vi "Follower.vi"   [LabVIEW 2016]
uses:
  <vilib>/NXT/Block Support/NXT_InputPort.ctl
  <vilib>/NXT/Block Support/NXT_TimerIndex.ctl
  <vilib>/NXT/Block Support/NXT_OutputPort.ctl
  <vilib>/NXT/Dual Mode Library/Sensors/EV3_Color_Reflect.vi
  <vilib>/NXT/NXTIO Xnodes/NXTIONodeSubVIs/NXTStopMotors.vi
  <vilib>/NXT/Dual Mode Library/Sensors/EV3_Ultrasonic_CM.vi
  <vilib>/NXT/NXTIO Xnodes/NXTIONodeSubVIs/NXTMoveMotors.vi
  <vilib>/NXT/Dual Mode Library/Display/drawText_Right.vi
  <vilib>/NXT/Dual Mode Library/Display/drawNumber.vi
  <vilib>/NXT/Dual Mode Library/Display/drawNumber_float.vi
  <vilib>/NXT/Dual Mode Library/Sensors/Touch_Pressed.vi
  <vilib>/NXT/Dual Mode Library/Display/drawText.vi
  <vilib>/NXT/Subs/LVHSConnector.ctl
  <vilib>/NXT/NXTIO Xnodes/AddressXNode/NXTIOAddress.xnode
  <vilib>/NXT/NXTIO Xnodes/NXTIOXNode/NXTIO.xnode
  <vilib>/NXT/LegoClasses/BrickReference/BrickReference.lvclass
types:
  T1 = typedef "NXT_TimerIndex.ctl" = u8
  T2 = typedef "LVHSConnector.ctl" = refnum<class "BrickReference.lvclass">
  T3 = typedef "NXT_InputPort.ctl" = u32
  T4 = typedef "NXT_OutputPort.ctl" = u8
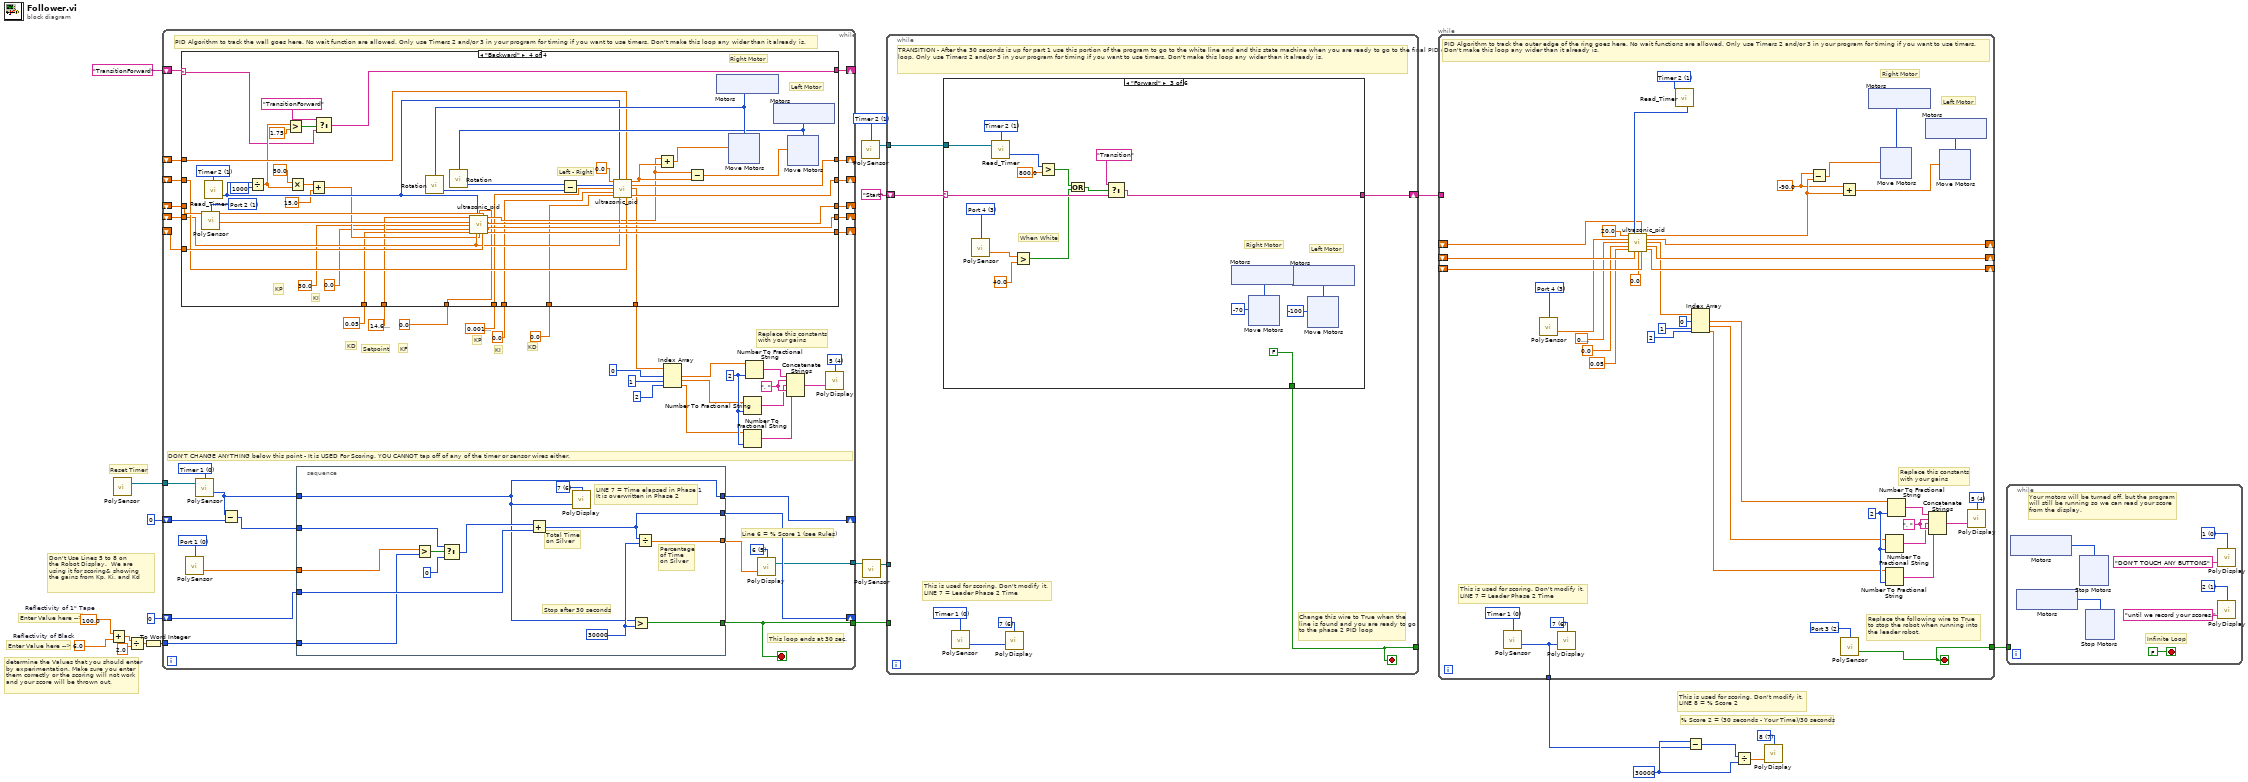
[diagram p0: block diagram]
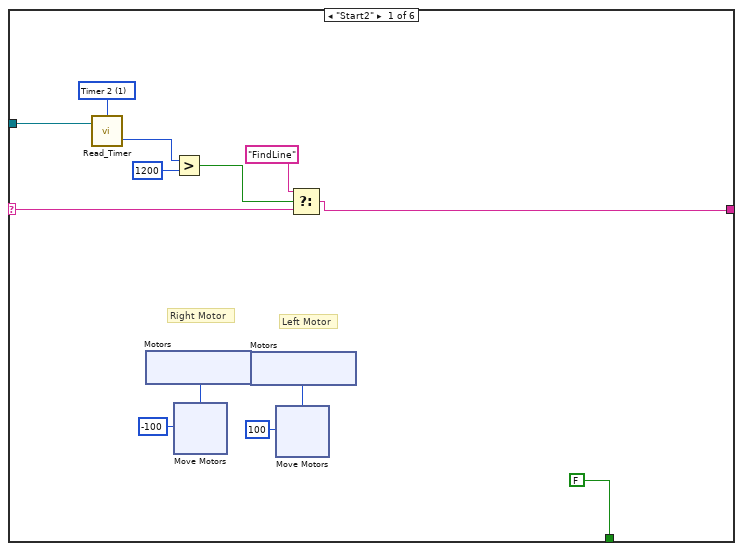
[diagram p2: hidden frame]
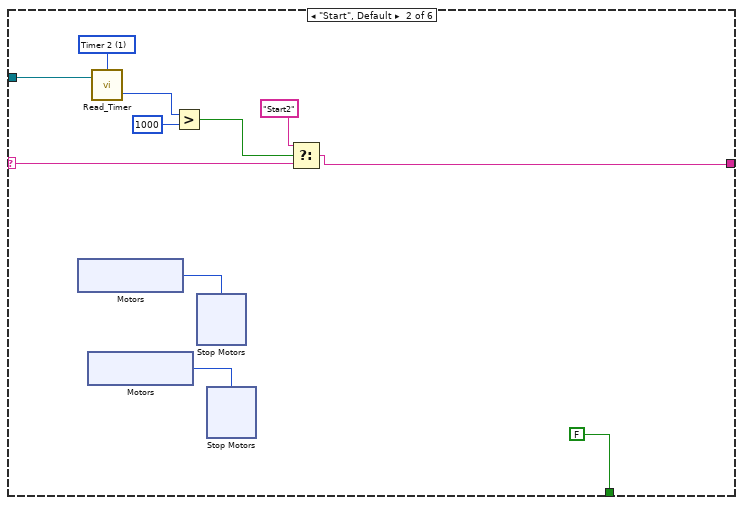
[diagram p3: hidden frame]
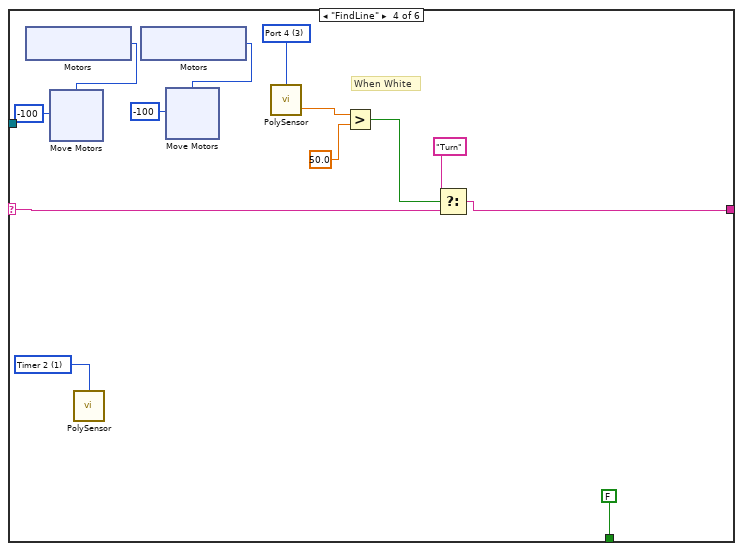
[diagram p4: hidden frame]
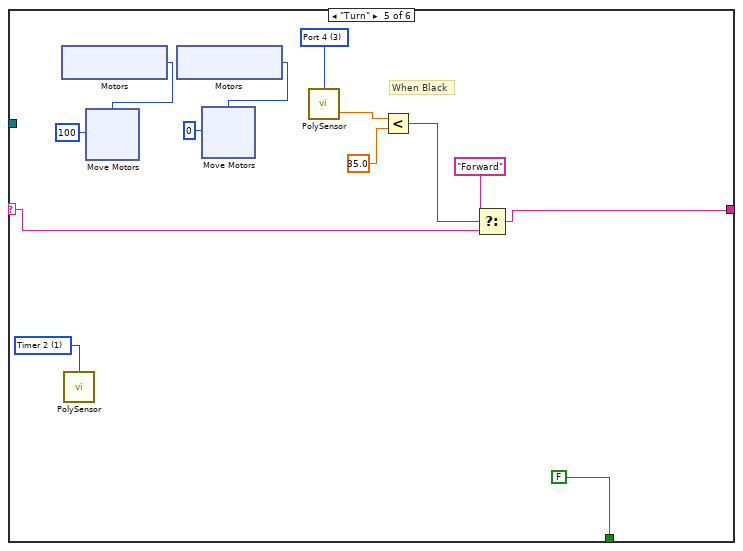
[diagram p5: hidden frame]
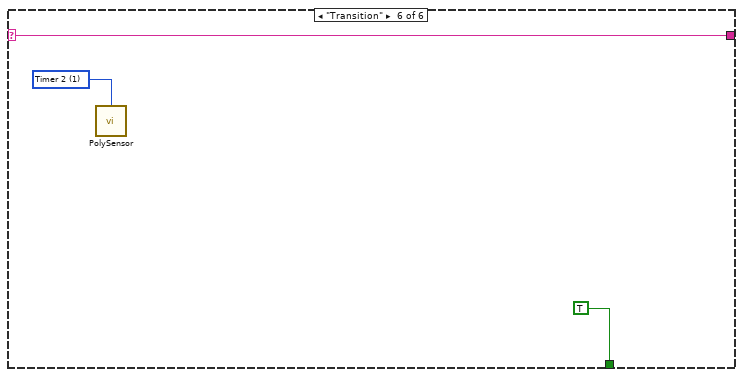
[diagram p6: hidden frame]
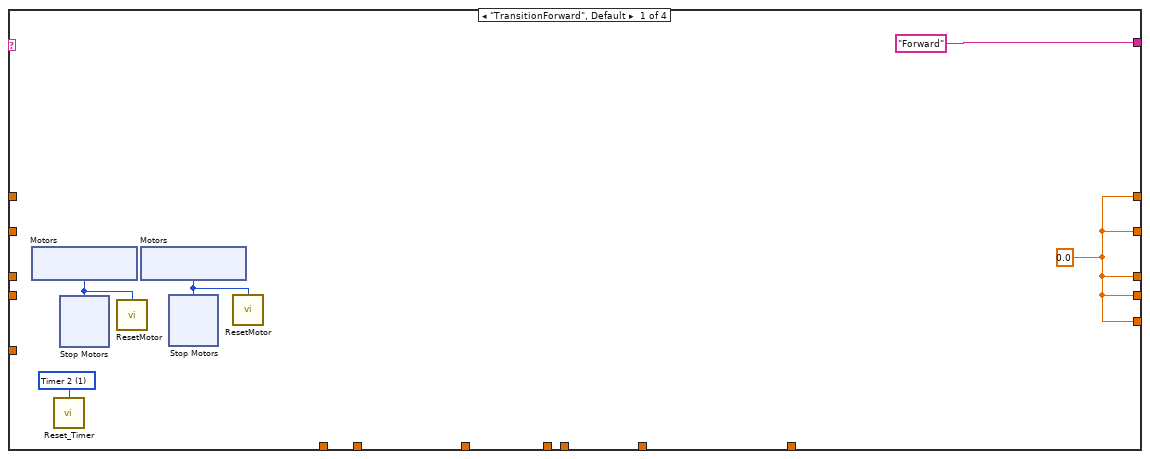
[diagram p7: hidden frame]
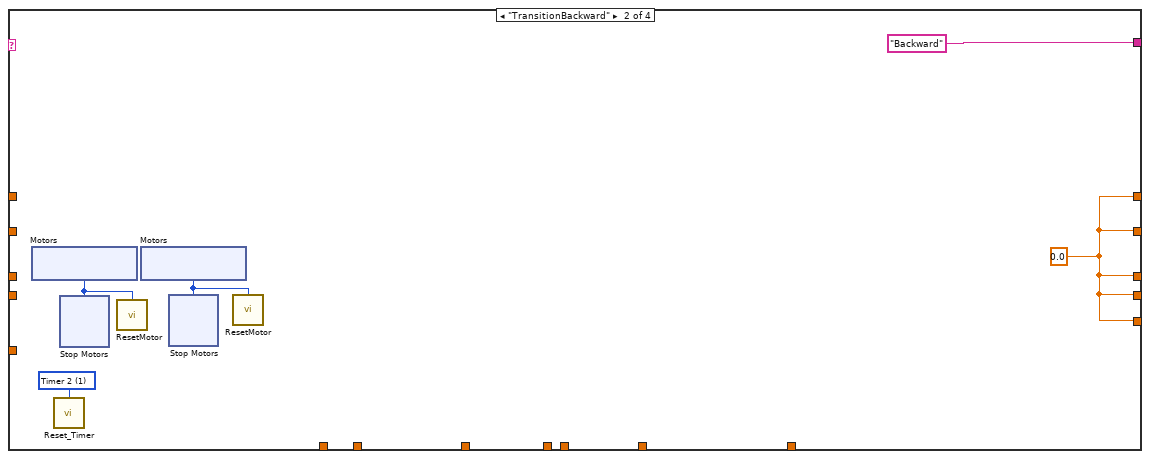
[diagram p8: hidden frame]
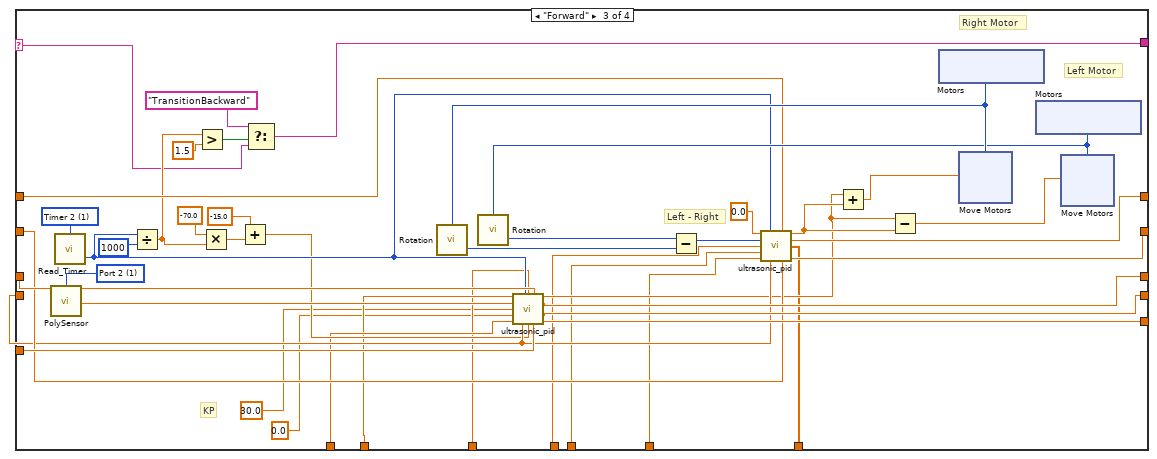
[diagram p9: hidden frame]
diagram:
  w1 = T1 1 items=["Timer 1", "Timer 2", "Timer 3"] ("Timer (Timer 1)")
  w7 = u32 30000 ("Value (msec)")
  w8 = i16 7 items=["1", "2", "3", "4", "5", "6", "7", "8", "9", "10", "11", "12"] ("Line")
  w14 = 6.0  # Reflectivity of Black
  w13 = 100.0  # Reflectivity of 1" Tape
  # "This is used for scoring. Don't modify it.\nLINE 8 = % Score 2"
  # "Don't Use Lines 5 to 8 on\nthe Robot Display.  We are \nusing it for scoring& showing \nthe gains from Kp, Ki, and Kd"
  # "% Score 2 = (30 seconds - Your Time)/30 seconds"
  # "Enter Value here -->"
  # "determine the Values that you should enter\nby experimentation. Make sure you enter \nthem correctly or the scoring will not work\nand your score will be thrown out."
  # "Enter Value here -->"
  # "Reset Timer"
  n1 = Add(x=w13, y=w14) -> (x+y=w12:dbl)
  n2 = call-poly <vilib>:"PolySensor.vi"() -> ("NXT/EV3"=w21:T2)  [unwired: 4 in]
  n3 = Divide(x=w12, y=2.0) -> (x/y=w11:dbl)
  n4 = To Word Integer(number=w11) -> (16bit integer=w18:i16)
  n5 = while {
    shift-right: [w66] -> _
    shift-left: i16 0 -> [w70]
    shift-right: [w67] -> _
    shift-left: i16 0 ("Value (msec)") -> [w69]
    tunnel: w21 -> [w65]
    tunnel: [w68] -> w20
    tunnel: w18 -> [w60]
    tunnel: [w56] -> w16
    shift-right: [w46] -> _
    shift-left: _ -> [w45]
    shift-right: [w47] -> _
    shift-left: _ -> [w44]
    shift-right: [w48] -> _
    shift-left: _ -> [w43]
    shift-right: [w42] -> _
    shift-left: _ -> [w40]
    shift-right: [w41] -> _
    shift-left: _ -> [w39]
    shift-right: [w37] -> _
    shift-left: "TransitionForward" -> [w38]
    stop <- w68 stop-if-true
    w52 = ", " ("string")
    w54 = i16 2 ("precision (6)")
    w55 = i16 4 items=["1", "2", "3", "4", "5", "6", "7", "8", "9", "10", "11", "12"] ("Line")
    w58 = i16 5 items=["1", "2", "3", "4", "5", "6", "7", "8", "9", "10", "11", "12"] ("Line")
    w62 = T3 0 items=["Port 1", "Port 2", "Port 3", "Port 4"] ("Port (Port 3)")
    w63 = T1 0 items=["Timer 1", "Timer 2", "Timer 3"] ("Timer (Timer 1)")
    # "KD"
    # "KI"
    # "KP"
    # "KD"
    # "KF"
    # "Setpoint"
    # "Replace this constants\nwith your gains"
    # "DON'T CHANGE ANYTHING below this point - It is USED For Scoring. YOU CANNOT tap off of any of the timer or sensor wires either."
    # "Line 6 = % Score 1 (see Rules)"
    # "This loop ends at 30 sec."
    # "PID Algorithm to track the wall goes here. No wait function are allowed. Only use Timers 2 and/or 3 in your program for timing if you want to use timers. Don't make this loop any wider than it already is."
    n6 = case shown="\"Backward\"" w38 {
      selector: w38 -> [_ _ w119 w182]
      tunnel: [w71 w88 w147 w207] -> w48
      tunnel: [w71 w88 w146 w206] -> w47
      tunnel: [w71 w88 w145 w205] -> w46
      tunnel: w45 -> [_ _ w144 w204]
      tunnel: w44 -> [_ _ w116 w176]
      tunnel: w43 -> [_ _ w143 w203]
      tunnel: [w71 w88 w135 w195] -> w42
      tunnel: [w71 w88 w134 w194] -> w41
      tunnel: w40 -> [_ _ w132 w192]
      tunnel: w39 -> [_ _ w131 w191]
      tunnel: ["Forward" ("t") "Backward" ("t") w117 w180] -> w37
      tunnel: 0.05 ("KD") -> [_ _ w113 w173]
      tunnel: sgl 0.0 ("KF") -> [_ _ w111 w172]
      tunnel: sgl 14.7 ("Setpoint") -> [_ _ w112 w171]
      tunnel: sgl 0.001 ("KP") -> [_ _ w110 w170]
      tunnel: 0.0 ("KI") -> [_ _ w109 w169]
      tunnel: 0.0 ("KD") -> [_ _ w108 w168]
      tunnel: [_ _ w107 w167] -> w30
      frame "TransitionForward", Default {
        w71 = sgl 0.0 ("Error")
        w75 = T1 1 items=["Timer 1", "Timer 2", "Timer 3"] ("Timer (Timer 1)")
        n7 = xnode "Motors"() -> ("Motor"=w74:T4)
        n8 = call <vilib>:"Reset_Timer.vi"("Timer (Timer 1)"=w75) -> ()  [unwired: 3 in, 1 out]
        n9 = xnode "Stop Motors"("Motors"=w74) -> ()  [unwired: 1 in, 1 out]
        n10 = call <vilib>:"ResetMotor.vi"("Port (All Ports)"=w74) -> ()  [unwired: 3 in, 1 out]
        n11 = xnode "Motors"() -> ("Motor"=w73:T4)
        n12 = xnode "Stop Motors"("Motors"=w73) -> ()  [unwired: 1 in, 1 out]
        n13 = call <vilib>:"ResetMotor.vi"("Port (All Ports)"=w73) -> ()  [unwired: 3 in, 1 out]
      }
      frame "TransitionBackward" {
        w88 = sgl 0.0 ("Error")
        w92 = T1 1 items=["Timer 1", "Timer 2", "Timer 3"] ("Timer (Timer 1)")
        n14 = xnode "Motors"() -> ("Motor"=w91:T4)
        n15 = call <vilib>:"Reset_Timer.vi"("Timer (Timer 1)"=w92) -> ()  [unwired: 3 in, 1 out]
        n16 = xnode "Stop Motors"("Motors"=w91) -> ()  [unwired: 1 in, 1 out]
        n17 = call <vilib>:"ResetMotor.vi"("Port (All Ports)"=w91) -> ()  [unwired: 3 in, 1 out]
        n18 = xnode "Motors"() -> ("Motor"=w90:T4)
        n19 = xnode "Stop Motors"("Motors"=w90) -> ()  [unwired: 1 in, 1 out]
        n20 = call <vilib>:"ResetMotor.vi"("Port (All Ports)"=w90) -> ()  [unwired: 3 in, 1 out]
      }
      frame "Forward" {
        w141 = T3 1 items=["Port 1", "Port 2", "Port 3", "Port 4"] ("Port (Port 1)")
        w148 = T1 1 items=["Timer 1", "Timer 2", "Timer 3"] ("Timer (Timer 1)")
        # "Left - Right"
        # "Left Motor"
        # "Right Motor"
        # "KP"
        n21 = call-poly <vilib>:"PolySensor.vi"("Port (Port 1)"=w141) -> ("Centimeters"=w142:sgl)  [unwired: 2 in, 1 out]
        n22 = call <vilib>:"Read_Timer.vi"("Timer (Timer 1)"=w148) -> ("Value (msec)"=w124:u32)  [unwired: 2 in, 1 out]
        n23 = Divide(x=w124, y=u32 1000) -> (x/y=w122:dbl)
        n24 = Greater?(x=w122, y=1.5) -> (0:w120:bool)
        n25 = Multiply(x=-70.0, y=w122) -> (x*y=w126:dbl)
        n26 = Add(x=-15.0, y=w126) -> (x+y=w114:dbl)
        n27 = Select(t="TransitionBackward", s=w120, f=w119) -> (s? t:f=w117:string)
        n28 = call "ultrasonic_pid.vi"("Setpoint"=w112, "Time"=w124, "KF"=w111, "Error"=w143, "Input"=w142, "KP"=sgl 30.0, "KI"=0.0, "KD"=w113, "Previous Time"=w116, "Feed Forward"=w114, "Accumulated Error"=w144) -> ("Output"=w115:dbl, "Error"=w147:sgl, "Current Time"=w146:dbl, "Accumulated Error"=w145:dbl)  [unwired: 1 out]
        n29 = xnode "Motors"() -> ("Motor"=w140:T4)
        n30 = call <vilib>:"Rotation.vi"("Port (Port A)"=w140) -> ("Angle of Rotation"=w138:i32)  [unwired: 2 in, 1 out]
        n31 = xnode "Motors"() -> ("Motor"=w139:T4)
        n32 = call <vilib>:"Rotation.vi"("Port (Port A)"=w139) -> ("Angle of Rotation"=w137:i32)  [unwired: 2 in, 1 out]
        n33 = Subtract(x=w137, y=w138) -> (x-y=w136:i32)
        n34 = call "ultrasonic_pid.vi"("Setpoint"=sgl 0.0, "Time"=w124, "Error"=w131, "Input"=w136, "KP"=w110, "KI"=w109, "KD"=w108, "Previous Time"=w116, "Accumulated Error"=w132) -> ("Output"=w130:dbl, "Error"=w134:sgl, "Gains"=w107:dbl[], "Accumulated Error"=w135:dbl)  [unwired: 2 in, 1 out]
        n35 = Add(x=w115, y=w130) -> (x+y=w129:dbl)
        n36 = Subtract(x=w115, y=w130) -> (x-y=w128:dbl)
        n37 = xnode "Move Motors"("Power/Speed 1"=w129, "Motors"=w140) -> ()  [unwired: 1 in, 1 out]
        n38 = xnode "Move Motors"("Power/Speed 1"=w128, "Motors"=w139) -> ()  [unwired: 1 in, 1 out]
      }
      frame "Backward" {
        w201 = T3 1 items=["Port 1", "Port 2", "Port 3", "Port 4"] ("Port (Port 1)")
        w208 = T1 1 items=["Timer 1", "Timer 2", "Timer 3"] ("Timer (Timer 1)")
        # "KI"
        # "KP"
        # "Left - Right"
        # "Left Motor"
        # "Right Motor"
        n39 = call-poly <vilib>:"PolySensor.vi"("Port (Port 1)"=w201) -> ("Centimeters"=w202:sgl)  [unwired: 2 in, 1 out]
        n40 = call <vilib>:"Read_Timer.vi"("Timer (Timer 1)"=w208) -> ("Value (msec)"=w187:u32)  [unwired: 2 in, 1 out]
        n41 = Divide(x=w187, y=u32 1000) -> (x/y=w185:dbl)
        n42 = Greater?(x=w185, y=1.75) -> (0:w183:bool)
        n43 = Multiply(x=50.0, y=w185) -> (x*y=w178:dbl)
        n44 = Add(x=w178, y=15.0 ("x")) -> (x+y=w175:dbl)
        n45 = Select(t="TransitionForward", s=w183, f=w182) -> (s? t:f=w180:string)
        n46 = call "ultrasonic_pid.vi"("Setpoint"=w171, "Time"=w187, "KF"=w172, "Error"=w203, "Input"=w202, "KP"=sgl 30.0, "KI"=0.0, "KD"=w173, "Previous Time"=w176, "Feed Forward"=w175, "Accumulated Error"=w204) -> ("Output"=w174:dbl, "Error"=w207:sgl, "Current Time"=w206:dbl, "Accumulated Error"=w205:dbl)  [unwired: 1 out]
        n47 = xnode "Motors"() -> ("Motor"=w200:T4)
        n48 = call <vilib>:"Rotation.vi"("Port (Port A)"=w200) -> ("Angle of Rotation"=w198:i32)  [unwired: 2 in, 1 out]
        n49 = xnode "Motors"() -> ("Motor"=w199:T4)
        n50 = call <vilib>:"Rotation.vi"("Port (Port A)"=w199) -> ("Angle of Rotation"=w197:i32)  [unwired: 2 in, 1 out]
        n51 = Subtract(x=w197, y=w198) -> (x-y=w196:i32)
        n52 = call "ultrasonic_pid.vi"("Setpoint"=sgl 0.0, "Time"=w187, "Error"=w191, "Input"=w196, "KP"=w170, "KI"=w169, "KD"=w168, "Previous Time"=w176, "Accumulated Error"=w192) -> ("Output"=w190:dbl, "Error"=w194:sgl, "Gains"=w167:dbl[], "Accumulated Error"=w195:dbl)  [unwired: 2 in, 1 out]
        n53 = Add(x=w174, y=w190) -> (x+y=w189:dbl)
        n54 = Subtract(x=w174, y=w190) -> (x-y=w188:dbl)
        n55 = xnode "Move Motors"("Power/Speed 1"=w189, "Motors"=w200) -> ()  [unwired: 1 in, 1 out]
        n56 = xnode "Move Motors"("Power/Speed 1"=w188, "Motors"=w199) -> ()  [unwired: 1 in, 1 out]
      }
    }
    n57 = call-poly <vilib>:"PolySensor.vi"("Port (Port 1)"=w62) -> ("Scaled Value"=w61:sgl)  [unwired: 2 in, 1 out]
    n58 = call-poly <vilib>:"PolySensor.vi"("NXT/EV3"=w65, "Timer (Timer 1)"=w63) -> ("Value (msec)"=w64:u32)  [unwired: 1 in, 1 out]
    n59 = Subtract(x=w64, y=w69) -> (x-y=w59:u32)
    n60 = stacked-sequence {
      tunnel: w70 -> [w237]
      tunnel: [w227] -> w57
      tunnel: w64 -> [w225]
      tunnel: [w236] -> w68
      tunnel: w61 -> [w231]
      tunnel: w59 -> [w233]
      tunnel: [w225] -> w67
      tunnel: [w229] -> w66
      tunnel: w60 -> [w230]
      frame #0 {
        w226 = i16 6 items=["1", "2", "3", "4", "5", "6", "7", "8", "9", "10", "11", "12"] ("Line")
        w228 = u32 30000 ("Value (msec)")
        # "LINE 7 = Time elapsed in Phase 1\nIt is overwritten in Phase 2"
        # "Percentage\nof Time\non Silver"
        # "Stop after 30 seconds"
        # "Total Time\non Silver"
        n61 = Greater?(x=w231, y=w230) -> (0:w234:bool)
        n62 = Select(t=w233, s=w234, f=i16 0) -> (s? t:f=w232:u32)
        n63 = Add(x=w232, y=w237) -> (x+y=w229:u32)
        n64 = call-poly <vilib>:"PolyDisplay.vi"("number"=w225, "Line"=w226) -> ()  [unwired: 2 in, 1 out]
        n65 = Greater?(x=w225, y=w228) -> (0:w236:bool)
        n66 = Divide(x=w229, y=w228) -> (x/y=w227:dbl)
      }
    }
    n67 = Index Array(array=w30, index #1=0 ("index"), index #2=1 ("index"), index #3=2 ("index")) -> (element #1=w29:dbl, element #2=w28:dbl, element #3=w27:dbl)
    n68 = Number To Fractional String(number=w28, precision (6)=w54) -> (F-format string=w51:string)  [unwired: 2 in]
    n69 = Number To Fractional String(number=w27, precision (6)=w54) -> (F-format string=w50:string)  [unwired: 2 in]
    n70 = Number To Fractional String(number=w29, precision (6)=w54) -> (F-format string=w53:string)  [unwired: 2 in]
    n71 = call-poly <vilib>:"PolyDisplay.vi"("number"=w57, "Line"=w58) -> ("NXT/EV3"=w56:T2)  [unwired: 2 in]
    n72 = Concatenate Strings(w53, w52, w51, w52, w50) -> (w49:string)
    n73 = call-poly <vilib>:"PolyDisplay.vi"("Text"=w49, "Line"=w55) -> ()  [unwired: 2 in, 1 out]
  }
  n74 = call-poly <vilib>:"PolySensor.vi"("Timer (Timer 1)"=w1) -> ("NXT/EV3"=w2:T2)  [unwired: 3 in]
  n75 = call-poly <vilib>:"PolySensor.vi"("NXT/EV3"=w16) -> ("NXT/EV3"=w15:T2)  [unwired: 3 in]
  n76 = while {
    tunnel: w20 -> [_]
    shift-right: [w243] -> w9
    shift-left: "Start" -> [w244]
    tunnel: w15 -> [_]
    tunnel: [w239] -> _
    tunnel: w2 -> [w238]
    stop <- w239 stop-if-true
    w240 = i16 6 items=["1", "2", "3", "4", "5", "6", "7", "8", "9", "10", "11", "12"] ("Line")
    w242 = T1 0 items=["Timer 1", "Timer 2", "Timer 3"] ("Timer (Timer 1)")
    # "This is used for scoring. Don't modify it.\nLINE 7 = Leader Phase 2 Time"
    # "Change this wire to True when the line is found and you are ready to go to the phase 2 PID loop"
    # "TRANSITION - After the 30 seconds is up for part 1 use this portion of the program to go to the white line and end this state machine when you are ready to go to the final PID control loop. Only use Timers 2 and/or 3 in your program for timing if you want to use timers. Don't make this loop any wider than it already is."
    n77 = case shown="\"Forward\"" w244 {
      selector: w244 -> [w253 w280 w310 w339 w367 w390]
      tunnel: [w252 w279 w309 w333 w366 w390] -> w243
      tunnel: [FALSE FALSE FALSE FALSE FALSE TRUE] -> w239
      tunnel: w238 -> [w256 w283 w313 _ _ _]
      frame "Start2" {
        w257 = T1 1 items=["Timer 1", "Timer 2", "Timer 3"] ("Timer (Timer 1)")
        # "Left Motor"
        # "Right Motor"
        n78 = call <vilib>:"Read_Timer.vi"("NXT/EV3"=w256, "Timer (Timer 1)"=w257) -> ("Value (msec)"=w255:u32)  [unwired: 1 in, 1 out]
        n79 = xnode "Motors"() -> ("Motor"=w248:T4)
        n80 = Greater?(x=w255, y=u32 1200) -> (0:w254:bool)
        n81 = xnode "Move Motors"("Power/Speed 1"=i8 -100, "Motors"=w248) -> ()  [unwired: 1 in, 1 out]
        n82 = xnode "Motors"() -> ("Motor"=w249:T4)
        n83 = xnode "Move Motors"("Power/Speed 1"=i8 100, "Motors"=w249) -> ()  [unwired: 1 in, 1 out]
        n84 = Select(t="FindLine", s=w254, f=w253) -> (s? t:f=w252:string)
      }
      frame "Start", Default {
        w284 = T1 1 items=["Timer 1", "Timer 2", "Timer 3"] ("Timer (Timer 1)")
        n85 = xnode "Motors"() -> ("Motor"=w276:T4)
        n86 = xnode "Motors"() -> ("Motor"=w275:T4)
        n87 = call <vilib>:"Read_Timer.vi"("NXT/EV3"=w283, "Timer (Timer 1)"=w284) -> ("Value (msec)"=w282:u32)  [unwired: 1 in, 1 out]
        n88 = Greater?(x=w282, y=u32 1000) -> (0:w281:bool)
        n89 = xnode "Stop Motors"("Motors"=w276) -> ()  [unwired: 1 in, 1 out]
        n90 = xnode "Stop Motors"("Motors"=w275) -> ()  [unwired: 1 in, 1 out]
        n91 = Select(t="Start2", s=w281, f=w280) -> (s? t:f=w279:string)
      }
      frame "Forward" {
        w300 = T3 3 items=["Port 1", "Port 2", "Port 3", "Port 4"] ("Port (Port 1)")
        w314 = T1 1 items=["Timer 1", "Timer 2", "Timer 3"] ("Timer (Timer 1)")
        # "When White"
        # "Left Motor"
        # "Right Motor"
        n92 = call-poly <vilib>:"PolySensor.vi"("Port (Port 1)"=w300) -> ("Scaled Value"=w301:sgl)  [unwired: 2 in, 1 out]
        n93 = call <vilib>:"Read_Timer.vi"("NXT/EV3"=w313, "Timer (Timer 1)"=w314) -> ("Value (msec)"=w311:u32)  [unwired: 1 in, 1 out]
        n94 = Greater?(x=w301, y=sgl 40.0) -> (0:w298:bool)
        n95 = Greater?(x=w311, y=800.0) -> (0:w299:bool)
        n96 = Or(x=w299, y=w298) -> (x .or. y?=w297:bool)
        n97 = Select(t="Transition", s=w297, f=w310) -> (s? t:f=w309:string)
        n98 = xnode "Motors"() -> ("Motor"=w305:T4)
        n99 = xnode "Move Motors"("Power/Speed 1"=i8 -70, "Motors"=w305) -> ()  [unwired: 1 in, 1 out]
        n100 = xnode "Motors"() -> ("Motor"=w306:T4)
        n101 = xnode "Move Motors"("Power/Speed 1"=i8 -100, "Motors"=w306) -> ()  [unwired: 1 in, 1 out]
      }
      frame "FindLine" {
        w331 = T1 1 items=["Timer 1", "Timer 2", "Timer 3"] ("Timer (Timer 1)")
        w338 = T3 3 items=["Port 1", "Port 2", "Port 3", "Port 4"] ("Port (Port 1)")
        # "When White"
        n102 = xnode "Motors"() -> ("Motor"=w343:T4)
        n103 = xnode "Move Motors"("Power/Speed 1"=i8 -100, "Motors"=w343) -> ()  [unwired: 1 in, 1 out]
        n104 = call-poly <vilib>:"PolySensor.vi"("Timer (Timer 1)"=w331) -> ()  [unwired: 3 in, 1 out]
        n105 = xnode "Motors"() -> ("Motor"=w342:T4)
        n106 = xnode "Move Motors"("Power/Speed 1"=i8 -100, "Motors"=w342) -> ()  [unwired: 1 in, 1 out]
        n107 = call-poly <vilib>:"PolySensor.vi"("Port (Port 1)"=w338) -> ("Scaled Value"=w337:sgl)  [unwired: 2 in, 1 out]
        n108 = Greater?(x=w337, y=sgl 50.0) -> (0:w335:bool)
        n109 = Select(t="Turn", s=w335, f=w339) -> (s? t:f=w333:string)
      }
      frame "Turn" {
        w360 = T1 1 items=["Timer 1", "Timer 2", "Timer 3"] ("Timer (Timer 1)")
        w364 = T3 3 items=["Port 1", "Port 2", "Port 3", "Port 4"] ("Port (Port 1)")
        # "When Black"
        n110 = xnode "Motors"() -> ("Motor"=w370:T4)
        n111 = call-poly <vilib>:"PolySensor.vi"("Timer (Timer 1)"=w360) -> ()  [unwired: 3 in, 1 out]
        n112 = xnode "Move Motors"("Power/Speed 1"=i8 100, "Motors"=w370) -> ()  [unwired: 1 in, 1 out]
        n113 = xnode "Motors"() -> ("Motor"=w369:T4)
        n114 = xnode "Move Motors"("Power/Speed 1"=i8 0, "Motors"=w369) -> ()  [unwired: 1 in, 1 out]
        n115 = call-poly <vilib>:"PolySensor.vi"("Port (Port 1)"=w364) -> ("Scaled Value"=w363:sgl)  [unwired: 2 in, 1 out]
        n116 = Less?(x=w363, y=sgl 35.0) -> (x < y?=w361:bool)
        n117 = Select(t="Forward", s=w361, f=w367) -> (s? t:f=w366:string)
      }
      frame "Transition" {
        w389 = T1 1 items=["Timer 1", "Timer 2", "Timer 3"] ("Timer (Timer 1)")
        n118 = call-poly <vilib>:"PolySensor.vi"("Timer (Timer 1)"=w389) -> ()  [unwired: 3 in, 1 out]
      }
    }
    n119 = call-poly <vilib>:"PolySensor.vi"("Timer (Timer 1)"=w242) -> ("Value (msec)"=w241:u32)  [unwired: 2 in, 1 out]
    n120 = call-poly <vilib>:"PolyDisplay.vi"("number"=w241, "Line"=w240) -> ()  [unwired: 2 in, 1 out]
  }
  n121 = while {
    tunnel: [w392] -> w10
    tunnel: w9 -> [_]
    tunnel: [w429] -> w6
    shift-right: [w414] -> _
    shift-left: _ -> [w408]
    shift-right: [w415] -> _
    shift-left: _ -> [w409]
    shift-right: [w416] -> _
    shift-left: _ -> [w411]
    stop <- w392 stop-if-true
    w393 = -90.0 ("y")
    w402 = T3 2 items=["Port 1", "Port 2", "Port 3", "Port 4"] ("Port (Port 1)")
    w407 = T3 3 items=["Port 1", "Port 2", "Port 3", "Port 4"] ("Port (Port 1)")
    w413 = T1 1 items=["Timer 1", "Timer 2", "Timer 3"] ("Timer (Timer 1)")
    w425 = ", " ("string")
    w427 = i16 2 ("precision (6)")
    w428 = i16 4 items=["1", "2", "3", "4", "5", "6", "7", "8", "9", "10", "11", "12"] ("Line")
    w430 = i16 6 items=["1", "2", "3", "4", "5", "6", "7", "8", "9", "10", "11", "12"] ("Line")
    w431 = T1 0 items=["Timer 1", "Timer 2", "Timer 3"] ("Timer (Timer 1)")
    # "Left Motor"
    # "Right Motor"
    # "Replace this constants\nwith your gains"
    # "This is used for scoring. Don't modify it.\nLINE 7 = Leader Phase 2 Time"
    # "PID Algorithm to track the outer edge of the ring goes here. No wait functions are allowed. Only use Timers 2 and/or 3 in your program for timing if you want to use timers.\nDon't make this loop any wider than it already is."
    # "Replace the following wire to True\nto stop the robot when running into \nthe leader robot."
    n122 = call-poly <vilib>:"PolySensor.vi"("Timer (Timer 1)"=w431) -> ("Value (msec)"=w429:u32)  [unwired: 2 in, 1 out]
    n123 = call-poly <vilib>:"PolySensor.vi"("Port (Port 1)"=w407) -> ("Scaled Value"=w406:sgl)  [unwired: 2 in, 1 out]
    n124 = call-poly <vilib>:"PolyDisplay.vi"("number"=w429, "Line"=w430) -> ()  [unwired: 2 in, 1 out]
    n125 = call <vilib>:"Read_Timer.vi"("Timer (Timer 1)"=w413) -> ("Value (msec)"=w412:u32)  [unwired: 2 in, 1 out]
    n126 = call "ultrasonic_pid.vi"("Setpoint"=sgl 20.0, "Time"=w412, "Error"=w408, "Input"=w406, "KP"=sgl 0.7, "KI"=0.0, "KD"=0.05, "Previous Time"=w409, "Feed Forward"=sgl 0.0, "Accumulated Error"=w411) -> ("Output"=w394:dbl, "Error"=w414:sgl, "Gains"=w401:dbl[], "Current Time"=w415:dbl, "Accumulated Error"=w416:dbl)  [unwired: 1 in]
    n127 = Index Array(array=w401, index #1=0 ("index"), index #2=1 ("index"), index #3=2 ("index")) -> (element #1=w397:dbl, element #2=w396:dbl, element #3=w395:dbl)
    n128 = Subtract(x=w393, y=w394) -> (x-y=w419:dbl)
    n129 = Add(x=w393, y=w394) -> (x+y=w418:dbl)
    n130 = call-poly <vilib>:"PolySensor.vi"("Port (Port 1)"=w402) -> ("Yes / No"=w392:bool)  [unwired: 2 in, 1 out]
    n131 = xnode "Motors"() -> ("Motor"=w421:T4)
    n132 = xnode "Move Motors"("Power/Speed 1"=w419, "Motors"=w421) -> ()  [unwired: 1 in, 1 out]
    n133 = Number To Fractional String(number=w396, precision (6)=w427) -> (F-format string=w424:string)  [unwired: 2 in]
    n134 = Number To Fractional String(number=w395, precision (6)=w427) -> (F-format string=w423:string)  [unwired: 2 in]
    n135 = Number To Fractional String(number=w397, precision (6)=w427) -> (F-format string=w426:string)  [unwired: 2 in]
    n136 = xnode "Motors"() -> ("Motor"=w420:T4)
    n137 = Concatenate Strings(w426, w425, w424, w425, w423) -> (w422:string)
    n138 = xnode "Move Motors"("Power/Speed 1"=w418, "Motors"=w420) -> ()  [unwired: 1 in, 1 out]
    n139 = call-poly <vilib>:"PolyDisplay.vi"("Text"=w422, "Line"=w428) -> ()  [unwired: 2 in, 1 out]
  }
  n140 = Subtract(x=w7, y=w6) -> (x-y=w5:u32)
  n141 = Divide(x=w5, y=w7) -> (x/y=w4:dbl)
  n142 = call-poly <vilib>:"PolyDisplay.vi"("number"=w4, "Line"=w8) -> ()  [unwired: 2 in, 1 out]
  n143 = while {
    tunnel: w10 -> [_]
    stop <- FALSE stop-if-true
    w448 = i16 1 items=["1", "2", "3", "4", "5", "6", "7", "8", "9", "10", "11", "12"] ("Line")
    w451 = i16 0 items=["1", "2", "3", "4", "5", "6", "7", "8", "9", "10", "11", "12"] ("Line")
    # "Your motors will be turned off, but the program\nwill still be running so we can read your score\nfrom the display."
    # "Infinite Loop"
    n144 = xnode "Motors"() -> ("Motor"=w453:T4)
    n145 = xnode "Motors"() -> ("Motor"=w452:T4)
    n146 = xnode "Stop Motors"("Motors"=w453) -> ()  [unwired: 1 in, 1 out]
    n147 = xnode "Stop Motors"("Motors"=w452) -> ()  [unwired: 1 in, 1 out]
    n148 = call-poly <vilib>:"PolyDisplay.vi"("Text"="DON'T TOUCH ANY BUTTONS", "Line"=w451) -> ()  [unwired: 2 in, 1 out]
    n149 = call-poly <vilib>:"PolyDisplay.vi"("Text"="until we record your scores.", "Line"=w448) -> ()  [unwired: 2 in, 1 out]
  }
